vi "one_of_n.vi"(5 "Reset":bool, 7 "Period length (Ts, sec)":dbl=1.0, 9 "Interval (decimate)":dbl=5.0) -> (2 "Now":bool)   [LabVIEW 2012]
panel:
  # "Though the general parameters are most naturally applied to point-by-point decimation, this can be applied to any one-out-of-n problem.  If a sample period in seconds is supplied then interval is also in seconds.  Interval need not be an integer, though values < 1 aren't useful.   If the default \"Period length\" of 1 is used, then we simply return true every \"Interval\" calls, where interval can still be a decimal.\n\nReset causes \"Now\" to be true on that call."
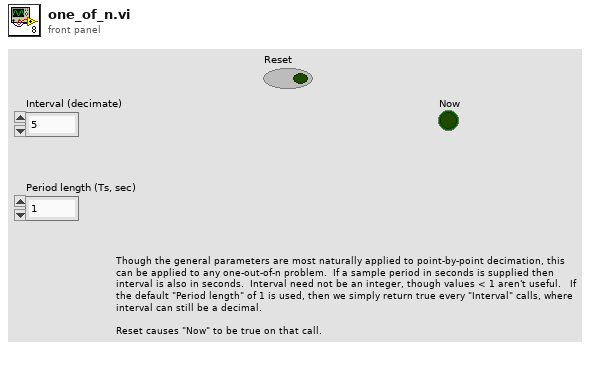
[diagram p1: front panel]
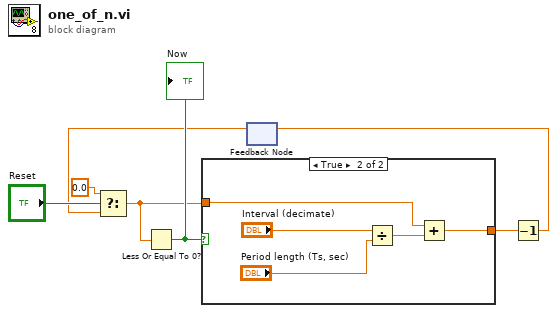
[diagram p0: block diagram]
diagram:
  n1 = feedback #1() -> (w2:dbl)  [unwired: 1 in]
  n2 = Select(t=0.0, s="Reset", f=w2) -> (s? t:f=w3:dbl)
  n3 = Less Or Equal To 0?(x=w3) -> (x <= 0?=w5:bool)
  "Now" <- w5
  n4 = case shown="True" w5 {
    tunnel: [w8 w10] -> w7
    tunnel: w3 -> [w8 w9]
    frame False {
    }
    frame True {
      n5 = Divide(x="Interval (decimate)", y="Period length (Ts, sec)") -> (x/y=w11:dbl)
      n6 = Add(x=w9, y=w11) -> (x+y=w10:dbl)
    }
  }
  n7 = Decrement(x=w7) -> (x-1=w6:dbl)
  n8 = feedback-in #1(w6) -> ()
